vi "Completed.vi"(8 "error in (no error)":errorcluster, 11 "TurnInstruction.lvclass":refnum<class "TurnInstruction.lvclass">) -> (0 "error out":errorcluster, 3 "Completed":bool)   [LabVIEW 2015, in "TurnInstruction.lvclass"]
uses:
  TurnInstruction.lvclass
  TurnInstruction.lvclass/TurnInstruction.ctl
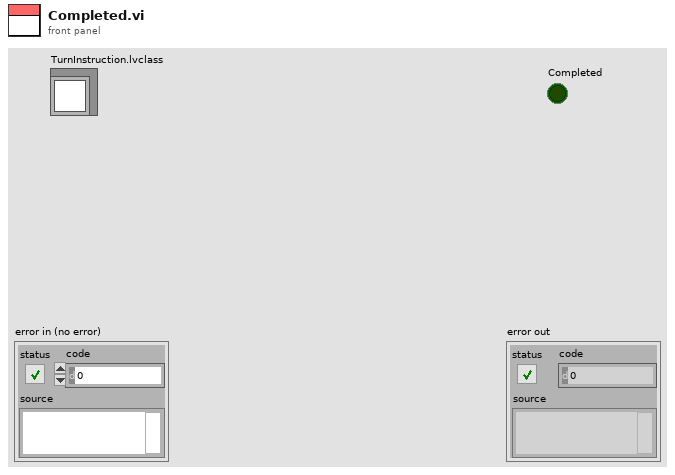
[diagram p1: front panel]
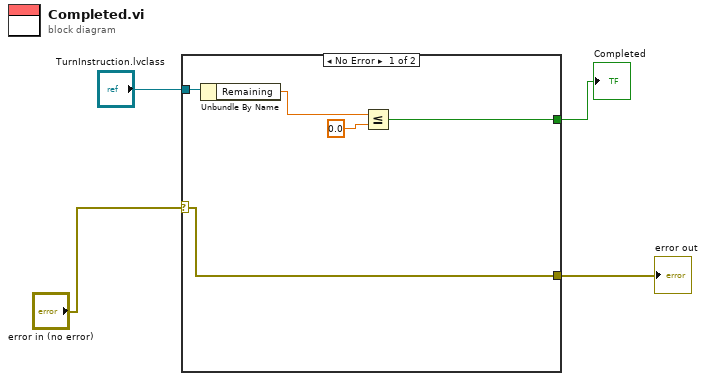
[diagram p0: block diagram]
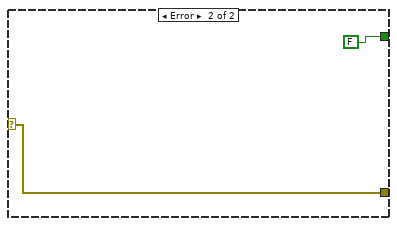
[diagram p2: hidden frame]
diagram:
  n1 = case shown="No Error" "error in (no error)" {
    selector: "error in (no error)" -> [w9 w11]
    tunnel: [w9 w11] -> w3
    tunnel: "TurnInstruction.lvclass" -> [w8 _]
    tunnel: [w5 FALSE] -> w1
    frame No Error {
      n2 = Unbundle By Name(w8) -> ("Remaining"=w7:dbl)
      n3 = Less Or Equal?(x=w7, y=0.0) -> (x <= y?=w5:bool)
    }
    frame Error {
    }
  }
  "error out" <- w3
  "Completed" <- w1
